vi "Test Protocols.vi"() -> ()   [LabVIEW 2013]
panel:
  in  "stop":bool
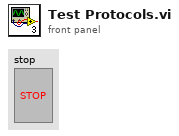
[diagram p1: front panel]
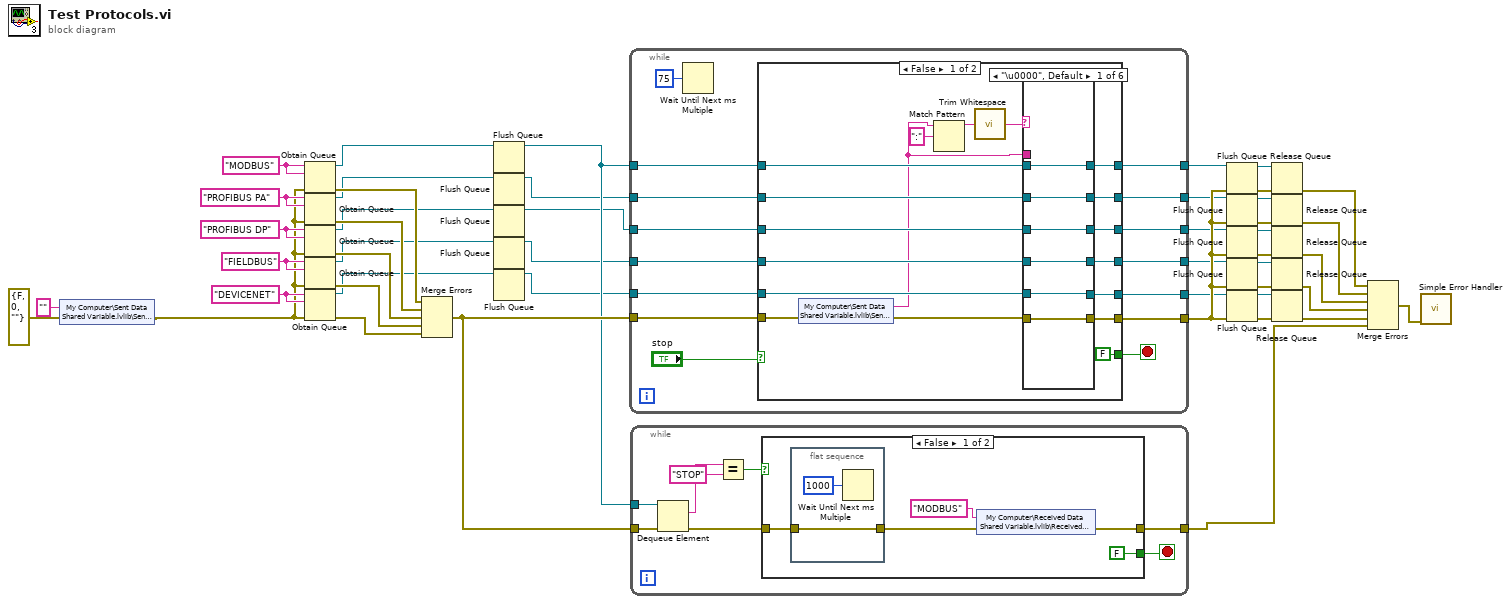
[diagram p0: block diagram]
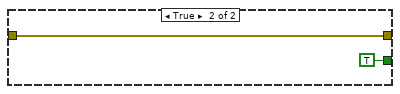
[diagram p2: hidden frame]
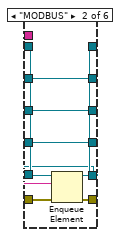
[diagram p3: hidden frame]
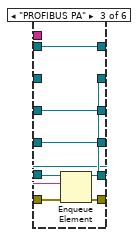
[diagram p4: hidden frame]
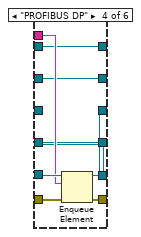
[diagram p5: hidden frame]
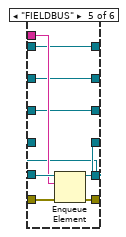
[diagram p6: hidden frame]
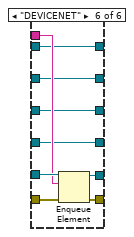
[diagram p7: hidden frame]
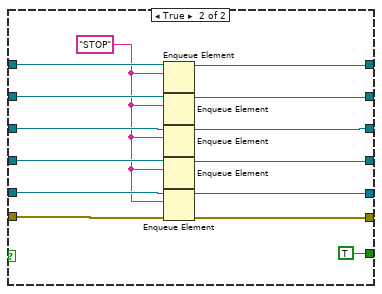
[diagram p8: hidden frame]
diagram:
  w43 = "DEVICENET" ("name (unnamed)")
  w44 = "FIELDBUS" ("name (unnamed)")
  w45 = "PROFIBUS DP" ("name (unnamed)")
  w46 = "PROFIBUS PA" ("name (unnamed)")
  w47 = "MODBUS" ("name (unnamed)")
  n1 = shared-variable "My Computer\\Sent Data Shared Variable.lvlib\\Sent Data"("" ("Sent Data"), error in=errorcluster {"status"=FALSE, "code"=0, "source"=""} ("error constant")) -> (error out=w2:errorcluster)
  n2 = Obtain Queue(name (unnamed)=w47, element data type=w47, error in (no error)=w2) -> (queue out=w13:refnum<queue>, error out=w42:errorcluster)  [unwired: 2 in, 1 out]
  n3 = Obtain Queue(name (unnamed)=w46, element data type=w46, error in (no error)=w2) -> (queue out=w12:refnum<queue>, error out=w41:errorcluster)  [unwired: 2 in, 1 out]
  n4 = Obtain Queue(name (unnamed)=w45, element data type=w45, error in (no error)=w2) -> (queue out=w11:refnum<queue>, error out=w40:errorcluster)  [unwired: 2 in, 1 out]
  n5 = Obtain Queue(name (unnamed)=w44, element data type=w44, error in (no error)=w2) -> (queue out=w10:refnum<queue>, error out=w39:errorcluster)  [unwired: 2 in, 1 out]
  n6 = Obtain Queue(name (unnamed)=w43, element data type=w43, error in (no error)=w2) -> (queue out=w9:refnum<queue>, error out=w38:errorcluster)  [unwired: 2 in, 1 out]
  n7 = Merge Errors(w42, w41, w40, w39, w38) -> (w15:errorcluster)
  n8 = Flush Queue(queue=w13) -> (queue out=w8:refnum<queue>)  [unwired: 1 in, 2 out]
  n9 = Flush Queue(queue=w12) -> (queue out=w7:refnum<queue>)  [unwired: 1 in, 2 out]
  n10 = Flush Queue(queue=w11) -> (queue out=w6:refnum<queue>)  [unwired: 1 in, 2 out]
  n11 = Flush Queue(queue=w10) -> (queue out=w5:refnum<queue>)  [unwired: 1 in, 2 out]
  n12 = Flush Queue(queue=w9) -> (queue out=w4:refnum<queue>)  [unwired: 1 in, 2 out]
  n13 = while {
    tunnel: w8 -> [w62]
    tunnel: w7 -> [w61]
    tunnel: w6 -> [w60]
    tunnel: w5 -> [w59]
    tunnel: w4 -> [w58]
    tunnel: w15 -> [w50]
    tunnel: [w57] -> w21
    tunnel: [w56] -> w20
    tunnel: [w55] -> w19
    tunnel: [w54] -> w18
    tunnel: [w53] -> w17
    tunnel: [w52] -> w16
    stop <- w48 stop-if-true
    n14 = Wait Until Next ms Multiple(millisecond multiple=u32 75) -> ()  [unwired: 1 out]
    n15 = case shown="False" "stop" {
      tunnel: w62 -> [w80 w143]
      tunnel: w61 -> [w79 w142]
      tunnel: w60 -> [w78 w141]
      tunnel: w59 -> [w77 w140]
      tunnel: w58 -> [w76 w139]
      tunnel: [w75 w144] -> w57
      tunnel: [w74 w138] -> w56
      tunnel: [w73 w137] -> w55
      tunnel: [w72 w136] -> w54
      tunnel: [w71 w135] -> w53
      tunnel: [w70 w134] -> w52
      tunnel: w50 -> [w69 w145]
      tunnel: [FALSE TRUE] -> w48
      frame False {
        n16 = shared-variable "My Computer\\Sent Data Shared Variable.lvlib\\Sent Data"(error in=w69) -> (w64:string, error out=w66:errorcluster)
        n17 = Match Pattern(string=w64, regular expression=":") -> (before substring=w68:string)  [unwired: 1 in, 3 out]
        n18 = call <vilib>:"Trim Whitespace.vi"("string"=w68) -> ("trimmed string"=w65:string)  [unwired: 1 in]
        n19 = case shown="\"\", Default" w65 {
          tunnel: w80 -> [w86 w95 w100 w109 w118 w127]
          tunnel: w64 -> [_ w94 w102 w110 w119 w128]
          tunnel: w79 -> [w85 w90 w101 w108 w117 w126]
          tunnel: w78 -> [w84 w89 w98 w111 w116 w125]
          tunnel: w77 -> [w83 w88 w97 w106 w120 w124]
          tunnel: w76 -> [w82 w87 w96 w105 w114 w129]
          tunnel: w66 -> [w81 w93 w104 w113 w122 w131]
          tunnel: [w81 w92 w103 w112 w121 w130] -> w75
          tunnel: [w86 w91 w100 w109 w118 w127] -> w74
          tunnel: [w85 w90 w99 w108 w117 w126] -> w73
          tunnel: [w84 w89 w98 w107 w116 w125] -> w72
          tunnel: [w83 w88 w97 w106 w115 w124] -> w71
          tunnel: [w82 w87 w96 w105 w114 w123] -> w70
          frame "\u0000", Default {
          }
          frame "MODBUS" {
            n20 = Enqueue Element(queue=w95, element=w94, error in (no error)=w93) -> (queue out=w91:refnum<queue>, error out=w92:errorcluster)  [unwired: 1 in, 1 out]
          }
          frame "PROFIBUS PA" {
            n21 = Enqueue Element(queue=w101, element=w102, error in (no error)=w104) -> (queue out=w99:refnum<queue>, error out=w103:errorcluster)  [unwired: 1 in, 1 out]
          }
          frame "PROFIBUS DP" {
            n22 = Enqueue Element(queue=w111, element=w110, error in (no error)=w113) -> (queue out=w107:refnum<queue>, error out=w112:errorcluster)  [unwired: 1 in, 1 out]
          }
          frame "FIELDBUS" {
            n23 = Enqueue Element(queue=w120, element=w119, error in (no error)=w122) -> (queue out=w115:refnum<queue>, error out=w121:errorcluster)  [unwired: 1 in, 1 out]
          }
          frame "DEVICENET" {
            n24 = Enqueue Element(queue=w129, element=w128, error in (no error)=w131) -> (queue out=w123:refnum<queue>, error out=w130:errorcluster)  [unwired: 1 in, 1 out]
          }
        }
      }
      frame True {
        w133 = "STOP" ("element")
        n25 = Enqueue Element(queue=w143, element=w133) -> (queue out=w138:refnum<queue>)  [unwired: 2 in, 2 out]
        n26 = Enqueue Element(queue=w142, element=w133) -> (queue out=w137:refnum<queue>)  [unwired: 2 in, 2 out]
        n27 = Enqueue Element(queue=w141, element=w133) -> (queue out=w136:refnum<queue>)  [unwired: 2 in, 2 out]
        n28 = Enqueue Element(queue=w140, element=w133) -> (queue out=w135:refnum<queue>)  [unwired: 2 in, 2 out]
        n29 = Enqueue Element(queue=w139, element=w133, error in (no error)=w145) -> (queue out=w134:refnum<queue>, error out=w144:errorcluster)  [unwired: 1 in, 1 out]
      }
    }
  }
  n30 = while {
    tunnel: w8 -> [w153]
    tunnel: w15 -> [w152]
    tunnel: [w147] -> w14
    stop <- w146 stop-if-true
    n31 = Dequeue Element(queue=w153, error in (no error)=w152) -> (element=w151:string, error out=w148:errorcluster)  [unwired: 1 in, 2 out]
    n32 = Equal?(x=w151, y="STOP") -> (x = y?=w149:bool)
    n33 = case shown="False" w149 {
      tunnel: w148 -> [w157 w161]
      tunnel: [w155 w161] -> w147
      tunnel: [FALSE TRUE] -> w146
      frame False {
        n34 = flat-sequence {
          tunnel: w157 -> [w159]
          tunnel: [w159] -> w156
          frame #0 {
            n35 = Wait Until Next ms Multiple(millisecond multiple=u32 1000) -> ()  [unwired: 1 out]
          }
        }
        n36 = shared-variable "My Computer\\Received Data Shared Variable.lvlib\\Received Data"("MODBUS" ("Received Data"), error in=w156) -> (error out=w155:errorcluster)
      }
      frame True {
      }
    }
  }
  n37 = Flush Queue(queue=w20, error in (no error)=w21) -> (queue out=w37:refnum<queue>, error out=w36:errorcluster)  [unwired: 1 out]
  n38 = Flush Queue(queue=w19, error in (no error)=w21) -> (queue out=w35:refnum<queue>, error out=w34:errorcluster)  [unwired: 1 out]
  n39 = Flush Queue(queue=w18, error in (no error)=w21) -> (queue out=w33:refnum<queue>, error out=w32:errorcluster)  [unwired: 1 out]
  n40 = Flush Queue(queue=w17, error in (no error)=w21) -> (queue out=w31:refnum<queue>, error out=w30:errorcluster)  [unwired: 1 out]
  n41 = Flush Queue(queue=w16, error in (no error)=w21) -> (queue out=w29:refnum<queue>, error out=w28:errorcluster)  [unwired: 1 out]
  n42 = Release Queue(queue=w37, error in (no error)=w36) -> (error out=w23:errorcluster)  [unwired: 1 in, 2 out]
  n43 = Release Queue(queue=w35, error in (no error)=w34) -> (error out=w24:errorcluster)  [unwired: 1 in, 2 out]
  n44 = Release Queue(queue=w33, error in (no error)=w32) -> (error out=w25:errorcluster)  [unwired: 1 in, 2 out]
  n45 = Release Queue(queue=w31, error in (no error)=w30) -> (error out=w26:errorcluster)  [unwired: 1 in, 2 out]
  n46 = Release Queue(queue=w29, error in (no error)=w28) -> (error out=w27:errorcluster)  [unwired: 1 in, 2 out]
  n47 = Merge Errors(w23, w24, w25, w26, w27, w14) -> (w22:errorcluster)
  n48 = call <vilib>:"Simple Error Handler.vi"("error in (no error)"=w22) -> ()  [unwired: 4 in, 5 out]
